vi "Get Desktop Window_KT.vi"() -> (3 "hWnd":u32)   [LabVIEW 2017, in "KTools.lvlib"]
doc: "<---------Get desktop window---------->\n\nReturns window handle of desktop"
uses:
  KTools.lvlib
  user32.dll
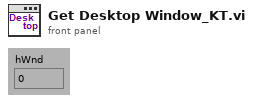
[diagram p1: front panel]
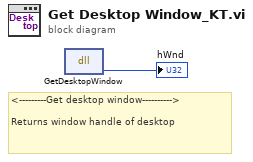
[diagram p0: block diagram]
diagram:
  # "<---------Get desktop window---------->\n\nReturns window handle of desktop"
  n1 = dll-call lib="user32.dll" fn="GetDesktopWindow"() -> (→"hWnd":u32)  [unwired: 3 in, 2 out]
